vi "Periodic Tasks.vi"(8 "error in (no error)":errorcluster) -> ()   [LabVIEW 2012]
doc: "This VI runs in parallel to other tasks. It can contain as many user-defined periodic loops as you need. These can carry out PID or other sorts of timed response."
uses:
  <vilib>/Rock Robotics/SystemInterfaces/Utilities/FPGA_UtilitiesLED Source.ctl
  <vilib>/Rock Robotics/SystemInterfaces/Utilities/FPGA_UtilitiesLED State.ctl
  <vilib>/Rock Robotics/WPI/CAN/Jaguar/SubVIs/WPI_CANJaguar_StatusSelect.ctl
  <vilib>/addons/Kinect/Skeleton Vertex Index.ctl
  <vilib>/addons/Kinect/SkeletonVertexTrackState.ctl
  Robot Global Data.vi
  <vilib>/addons/control/pid/pid.llb/PID (DBL).vi
  <vilib>/Rock Robotics/WPI/Joystick/WPI_JoystickGetSetRefNum.vi
  <vilib>/addons/control/pid/NI_PID_pid.lvlib
panel:
  in  "Kinect Drive?":bool
  in  "Kinect?":bool
  in  "Constant":dbl=-0.02
  in  "Not PID?":bool=TRUE
  in  "PID gains":T1={"proportional gain (Kc)"=1.0, "integral time (Ti, min)"=0.01, "derivative time (Td, min)"=0.0} {"derivative time (Td, min)" format="%.3f"; "integral time (Ti, min)" format="%.3f"; "proportional gain (Kc)" format="%.3f"}
  in  "c":dbl
  in  "b":dbl
  in  "a":dbl
  in  "Set Shooter speed":dbl
  in  "Linear":bool=TRUE
  in  "m":dbl=0.059
  in  "b":dbl=-0.047
  in  "Straight Add":dbl=20.0
  in  "Spin":dbl=0.5
  out "output":dbl format="%.2f"
  out "Set Speed":dbl
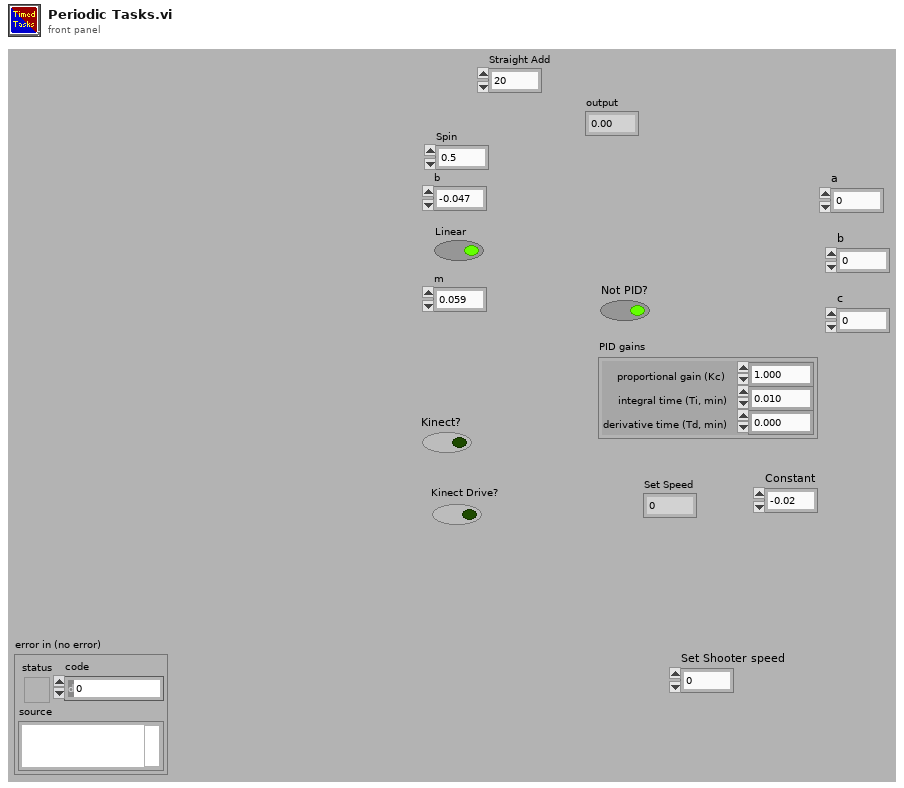
[diagram p1: front panel]
types:
  T1 = cluster{"proportional gain (Kc)":dbl, "integral time (Ti, min)":dbl, "derivative time (Td, min)":dbl}
  T2 = typedef "WPI_ServoDeviceRef.ctl" = cluster{"DeviceStatus":errorcluster, "Digital Module":T3, "PWM Channel":T4, "DeadBand":T5}
  T3 = typedef "FPGA_TypedefDigitalModule.ctl" = enum16{"Digital Module 1", "Digital Module 2"}
  T4 = typedef "FPGA_DIOPWMChannel.ctl" = enum8{"PWM 1", "PWM 2", "PWM 3", "PWM 4", "PWM 5", "PWM 6", "PWM 7", "PWM 8", "PWM 9", "PWM 10", "Invalid"}
  T5 = typedef "WPI_PWMDeadband.ctl" = cluster{"Name":string, "maxPositivePwm":i32, "minPositivePwm":i32, "centerPwm":i32, "maxNegativePwm":i32, "minNegativePwm":i32, "angularRange":u16}
  T6 = typedef "WPI_GyroDevRef.ctl" = cluster{"DevStatus":errorcluster, "Analog Module":T7, "Analog Channel":T8, "Offset":dbl, "Gain (VoltsPerDegree/Second)":dbl}
  T7 = typedef "FPGA_TypedefAnalogModule.ctl" = enum16{"Analog Module 1", "Analog Module 2"}
  T8 = typedef "FPGA_AIChannel.ctl" = enum8{"AI 1", "AI 2", "AI 3", "AI 4", "AI 5", "AI 6", "AI 7", "AI 8", "Invalid"}
  T9 = typedef "WPI_JoystickDevRef.ctl" = cluster{"Device":T10}
  T10 = typedef "WPI_JoystickDeviceEnum.ctl" = enum16{"USB 1", "USB 2", "USB 3", "USB 4", "Kinect 1", "Kinect 2"}
  T11 = typedef "WPI_MotorControlDeviceRef.ctl" = cluster{"DeviceStatus":errorcluster, "Type":enum16{"PWM", "CAN"}, "PWM":cluster{"Digital Module":T3, "PWM Channel":T4, "DeadBand":T5}, "CAN":cluster{"Device Number":u8, "Control Mode":T12, "Semaphore":T13, "Max Vout":dbl}, "Invert":bool, "TransformRef":T14, "InvTransformRef":T14}
  T12 = typedef "WPI_CANJaguar_ControlMode.ctl" = enum8{"Percent VBus", "Current", "Speed", "Position", "Voltage"}
  T13 = typedef "Semaphore RefNum" = refnum<k1>
  T14 = typedef "WPI_PWMTransform_ConPane.ctl" = refnum<vi>
  T15 = typedef "WPI_CANJaguar_StatusSelect.ctl" = enum16{"Output Percent VBus", "Output Voltage", "Bus Voltage", "Current", "Temperature", "Position", "Speed", "Limit Switches", "Faults", "Fault Counters", "Power Cycle"}
  T16 = typedef "Skeleton Vertex Index.ctl" = i32
  T17 = typedef "SkeletonVertexTrackState.ctl" = enum32{"NotTracked", "Inferred", "Tracked"}
  T18 = typedef "WPI_CANJaguar_Status.ctl" = cluster{"Output Percent VBus":dbl, "Output Voltage":dbl, "Bus Voltage":dbl, "Current":dbl, "Temperature":dbl, "Position":dbl, "Speed":dbl, "Limits":cluster{"Forward Limit":bool, "Reverse Limit":bool, "Forward Soft Limit":bool, "Reverse Soft Limit":bool, "Sticky Forward Limit":bool, "Sticky Reverse Limit":bool, "Sticky Forward Soft Limit":bool, "Sticky Reverse Soft Limit":bool}, "Faults":cluster{"Current Fault":bool, "Temperature Fault":bool, "Bus Voltage Fault":bool, "Gate Driver Fault":bool, "Comm Fault":bool}, "Fault Counters":cluster{"Current Faults":u8, "Temperature Faults":u8, "Bus Voltage Faults":u8, "Gate Driver Faults":u8, "Comm Faults":u8, "CAN Status":u8, "CAN RX Errors":u8, "CAN TX Errors":u8}, "Power Cycle":bool}
  T19 = cluster{cluster{"Left":dbl, "Top":dbl, "Right":dbl, "Bottom":dbl}, dbl[]}[]
  T20 = cluster{cluster{dbl, dbl, dbl}, cluster{"Right":dbl, "Left":dbl, "Bottom":dbl, "Top":dbl}}
  T21 = cluster{"Right":dbl, "Left":dbl, "Bottom":dbl, "Top":dbl}
  T22 = cluster{"axis 1 (x)":dbl, "axis 2 (y)":dbl, "axis 3 (throttle)":dbl, "axis 4":dbl, "axis 5":dbl, "axis 6":dbl}
  T23 = typedef "WPI_JoystickButtonState.ctl" = cluster{"Button 1":bool, "Button 2":bool, "Button 3":bool, "Button 4":bool, "Button 5":bool, "Button 6":bool, "Button 7":bool, "Button 8":bool, "Button 9":bool, "Button 10":bool, "Button 11":bool, "Button 12":bool}
  T24 = typedef "FPGA_UtilitiesLED State.ctl" = enum16{"Off", "On", "Toggle"}
  T25 = typedef "FPGA_UtilitiesLED Source.ctl" = enum16{"User LED", "FPGA LED"}
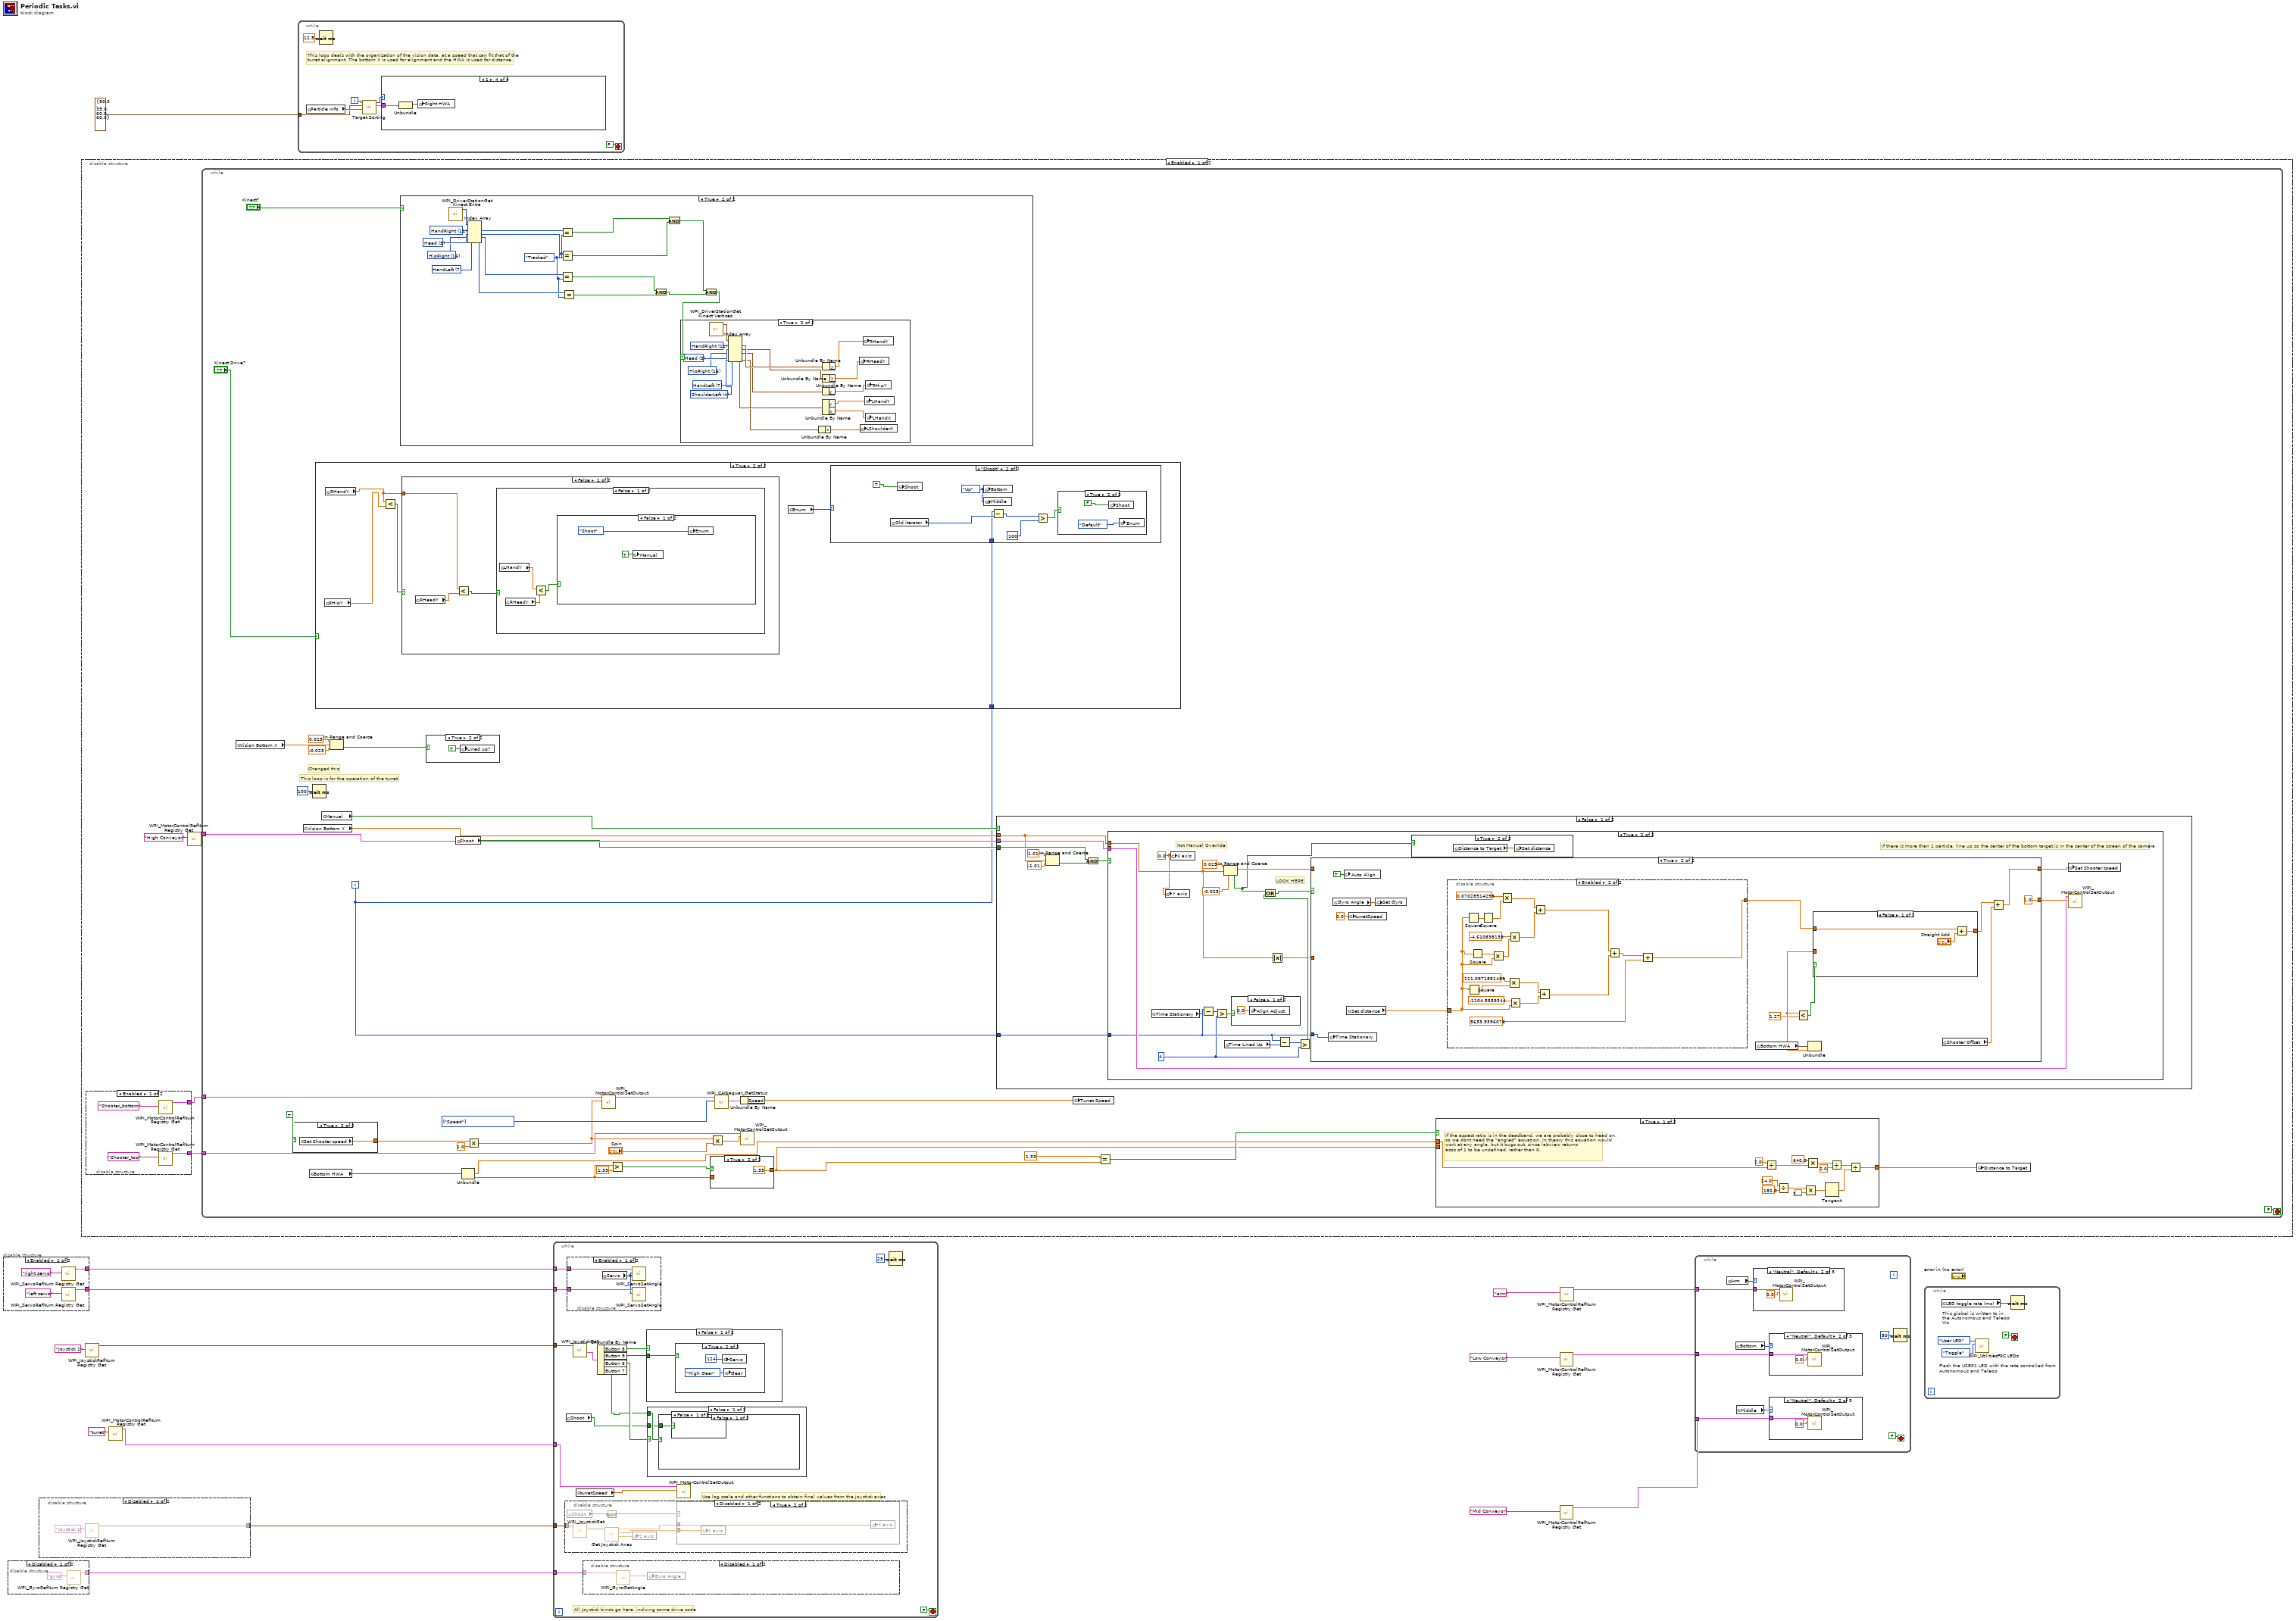
[diagram p0: block diagram]
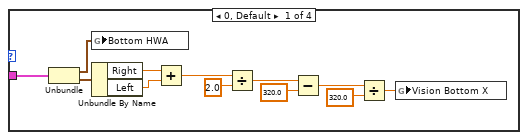
[diagram p3: hidden frame]
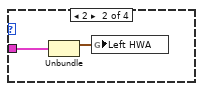
[diagram p4: hidden frame]
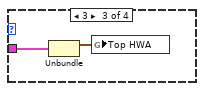
[diagram p5: hidden frame]
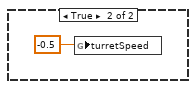
[diagram p11: hidden frame]
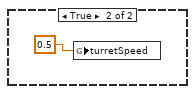
[diagram p12: hidden frame]
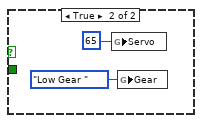
[diagram p15: hidden frame]
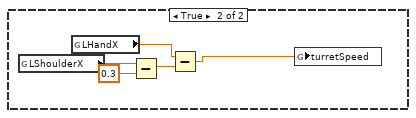
[diagram p19: hidden frame]
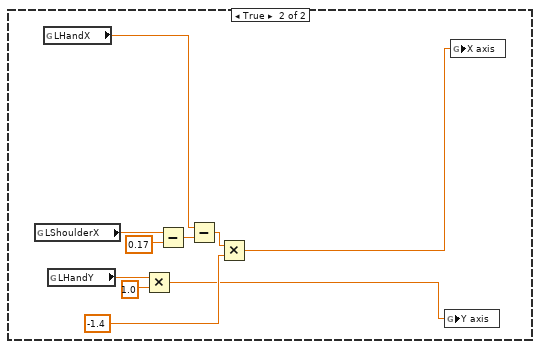
[diagram p20: hidden frame]
diagram:
  n1 = disable-structure shown="Enabled" {
    disable-tunnel: [w17 _] -> w9
    disable-tunnel: [w16 _] -> w8
    frame Enabled {
      n2 = call <vilib>:"WPI_ServoRefNum Registry Get.vi"("refnum name"="right servo") -> ("ServoDeviceRef"=w17:T2)  [unwired: 9 in, 1 out]
      n3 = call <vilib>:"WPI_ServoRefNum Registry Get.vi"("refnum name"="left servo") -> ("ServoDeviceRef"=w16:T2)  [unwired: 9 in, 1 out]
    }
    frame Disabled {
    }
  }
  n4 = disable-structure shown="Disabled" {
    disable-tunnel: [w21 _] -> w11
    frame Disabled {
      n5 = call <vilib>:"WPI_GyroRefNum Registry Get.vi"("refnum name"="gyro") -> ("GyroDevRef"=w21:T6)  [unwired: 9 in, 1 out]
    }
    frame Enabled {
    }
  }
  n6 = disable-structure shown="Disabled" {
    disable-tunnel: [w22 _] -> w12
    frame Disabled {
      n7 = call <vilib>:"WPI_JoystickRefNum Registry Get.vi"("refnum name"="Joystick 1") -> ("JoystickDevRef"=w22:T9)  [unwired: 9 in, 1 out]
    }
    frame Enabled {
    }
  }
  n8 = disable-structure shown="Enabled" {
    frame Enabled {
      n9 = disable-structure shown="Enabled" {
        disable-tunnel: [w31 _] -> w27
        disable-tunnel: [w30 _] -> w26
        frame Enabled {
          n10 = call <vilib>:"WPI_MotorControlRefNum Registry Get.vi"("refnum name"="Shooter_bottom") -> ("MotorControlDevRef"=w30:T11)  [unwired: 9 in, 1 out]
          n11 = call <vilib>:"WPI_MotorControlRefNum Registry Get.vi"("refnum name"="Shooter_top") -> ("MotorControlDevRef"=w31:T11)  [unwired: 9 in, 1 out]
        }
        frame Disabled {
        }
      }
      n12 = call <vilib>:"WPI_MotorControlRefNum Registry Get.vi"("refnum name"="High Conveyor") -> ("MotorControlDevRef"=w24:T11)  [unwired: 9 in, 1 out]
      n13 = while {
        tunnel: w27 -> [w63]
        tunnel: w26 -> [w62]
        tunnel: w24 -> [w39]
        i -> [w33]
        stop <- FALSE stop-if-true
        w58 = T15[] [enum."Speed"] items=["Output Percent VBus", "Output Voltage", "Bus Voltage", "Current", "Temperature", "Position", "Speed", "Limit Switches", "Faults", "Fault Counters", "Power Cycle"] ("Status Select")
        # "Changed this"
        # "This loop is for the operation of the turret."
        n14 = global read "Robot Global Data.vi" "Vision Bottom X"() -> (w43:dbl)
        n15 = case shown="True" TRUE {
          tunnel: ["Set Shooter speed" w145] -> w55
          frame False {
          }
          frame True {
            n16 = global read "Robot Global Data.vi" "Set Shooter speed"() -> (w145:dbl)
          }
        }
        n17 = global read "Robot Global Data.vi" "Vision Bottom X"() -> (w37:dbl)
        n18 = global read "Robot Global Data.vi" "Bottom HWA"() -> (w50:cluster{dbl, dbl, dbl})
        n19 = Wait (ms)(milliseconds to wait=u32 100) -> ()  [unwired: 1 out]
        n20 = case shown="True" "Kinect Drive?" {
          tunnel: w33 -> [_ w69]
          frame False {
          }
          frame True {
            n21 = global read "Robot Global Data.vi" "RHipY"() -> (w68:dbl)
            n22 = global read "Robot Global Data.vi" "RHandY"() -> (w66:dbl)
            n23 = Less?(x=w66, y=w68) -> (x < y?=w67:bool)
            n24 = case shown="False" w67 {
              tunnel: w66 -> [w73 _]
              frame False {
                n25 = global read "Robot Global Data.vi" "RHeadY"() -> (w72:dbl)
                n26 = Less?(x=w73, y=w72) -> (x < y?=w71:bool)
                n27 = case shown="False" w71 {
                  frame False {
                    n28 = global read "Robot Global Data.vi" "LHandY"() -> (w75:dbl)
                    n29 = global read "Robot Global Data.vi" "RHeadY"() -> (w74:dbl)
                    n30 = Less?(x=w75, y=w74) -> (x < y?=w76:bool)
                    n31 = case shown="False" w76 {
                      frame False {
                        n32 = global write "Robot Global Data.vi" "Manual"(TRUE ("Manual")) -> ()
                        n33 = global write "Robot Global Data.vi" "Enum"(enum16{"Default", "Shoot"}."Shoot" ("Enum")) -> ()
                      }
                      frame True {
                        n34 = global read "Robot Global Data.vi" "LShoulderX"() -> (w83:dbl)
                        n35 = global read "Robot Global Data.vi" "LHandX"() -> (w82:dbl)
                        n36 = Subtract(x=w83, y=0.3) -> (x-y=w80:dbl)
                        n37 = Subtract(x=w82, y=w80) -> (x-y=w81:dbl)
                        n38 = global write "Robot Global Data.vi" "turretSpeed"(w81) -> ()
                      }
                    }
                  }
                  frame True {
                    n39 = global read "Robot Global Data.vi" "LShoulderX"() -> (w87:dbl)
                    n40 = global read "Robot Global Data.vi" "LHandX"() -> (w93:dbl)
                    n41 = global read "Robot Global Data.vi" "LHandY"() -> (w92:dbl)
                    n42 = Multiply(x=w92, y=1.0) -> (x*y=w90:dbl)
                    n43 = Subtract(x=w87, y=0.17 ("x")) -> (x-y=w85:dbl)
                    n44 = Subtract(x=w93, y=w85) -> (x-y=w88:dbl)
                    n45 = Multiply(x=w88, y=-1.4) -> (x*y=w86:dbl)
                    n46 = global write "Robot Global Data.vi" "Y axis"(w90) -> ()
                    n47 = global write "Robot Global Data.vi" "X axis"(w86) -> ()
                  }
                }
              }
              frame True {
                w94 = 0.0 ("X axis")
                n48 = global write "Robot Global Data.vi" "X axis"(w94) -> ()
                n49 = global write "Robot Global Data.vi" "Y axis"(0.0 ("Y axis")) -> ()
                n50 = global write "Robot Global Data.vi" "Shoot"(FALSE) -> ()
                n51 = global write "Robot Global Data.vi" "turretSpeed"(w94) -> ()
                n52 = global write "Robot Global Data.vi" "Enum"(enum16{"Default", "Shoot"}."Default" ("Enum")) -> ()
              }
            }
            n53 = global read "Robot Global Data.vi" "Enum"() -> (w70:enum16{"Default", "Shoot"})
            n54 = case shown="\"Shoot\"" w70 {
              tunnel: w69 -> [w100 w103]
              frame "Default", Default {
                w99 = enum16{"Up", "Neutral", "Down"}."Neutral" ("Bottom")
                n55 = global write "Robot Global Data.vi" "Set Shooter speed"(0.0 ("Set Shooter speed")) -> ()
                n56 = global write "Robot Global Data.vi" "Old iterator"(w100) -> ()
                n57 = global write "Robot Global Data.vi" "Bottom"(w99) -> ()
                n58 = global write "Robot Global Data.vi" "Bottom"(w99) -> ()
              }
              frame "Shoot" {
                w101 = enum16{"Up", "Neutral", "Down"}."Up" ("Bottom")
                n59 = global read "Robot Global Data.vi" "Old iterator"() -> (w104:i8)
                n60 = global write "Robot Global Data.vi" "Shoot"(TRUE) -> ()
                n61 = global write "Robot Global Data.vi" "Bottom"(w101) -> ()
                n62 = global write "Robot Global Data.vi" "Middle"(w101) -> ()
                n63 = Subtract(x=w103, y=w104) -> (x-y=w102:i32)
                n64 = Greater?(x=w102, y=u32 100 ("milliseconds to wait")) -> (0:w105:bool)
                n65 = case shown="True" w105 {
                  frame False {
                  }
                  frame True {
                    n66 = global write "Robot Global Data.vi" "Shoot"(FALSE) -> ()
                    n67 = global write "Robot Global Data.vi" "Enum"(enum16{"Default", "Shoot"}."Default" ("Enum")) -> ()
                  }
                }
              }
            }
          }
        }
        n68 = global read "Robot Global Data.vi" "Manual"() -> (w35:bool)
        n69 = In Range and Coerce(upper limit=0.025, x=w43, lower limit=-0.025) -> (In Range?=w40:bool)  [unwired: 1 out]
        n70 = case shown="True" "Kinect?" {
          frame False {
          }
          frame True {
            w118 = T16 7 items=["HipCenter", "Spine", "ShoulderCenter", "Head", "ShoulderLeft", "ElbowLeft", "WristLeft", "HandLeft", "ShoulderRight", "ElbowRight", "WristRight", "HandRight", "HipLeft", "KneeLeft", "AnkleLeft", "FootLeft", "HipRight", "KneeRight", "AnkleRight", "FootRight"] ("Skeleton Joints")
            w119 = T16 16 items=["HipCenter", "Spine", "ShoulderCenter", "Head", "ShoulderLeft", "ElbowLeft", "WristLeft", "HandLeft", "ShoulderRight", "ElbowRight", "WristRight", "HandRight", "HipLeft", "KneeLeft", "AnkleLeft", "FootLeft", "HipRight", "KneeRight", "AnkleRight", "FootRight"] ("Skeleton Joints")
            w123 = T16 3 items=["HipCenter", "Spine", "ShoulderCenter", "Head", "ShoulderLeft", "ElbowLeft", "WristLeft", "HandLeft", "ShoulderRight", "ElbowRight", "WristRight", "HandRight", "HipLeft", "KneeLeft", "AnkleLeft", "FootLeft", "HipRight", "KneeRight", "AnkleRight", "FootRight"] ("Skeleton Joints")
            w115 = SkeletonVertexTrackState."Tracked" ("element")
            w125 = T16 11 items=["HipCenter", "Spine", "ShoulderCenter", "Head", "ShoulderLeft", "ElbowLeft", "WristLeft", "HandLeft", "ShoulderRight", "ElbowRight", "WristRight", "HandRight", "HipLeft", "KneeLeft", "AnkleLeft", "FootLeft", "HipRight", "KneeRight", "AnkleRight", "FootRight"] ("Skeleton Joints")
            n71 = call <vilib>:"WPI_DriverStationGet Kinect Extra.vi"() -> ("Skeleton Tracking State"=w126:T17[])  [unwired: 7 in, 4 out]
            n72 = Index Array(array=w126, index #1=w125, index #2=w123, index #3=w119, index #4=w118) -> (element #1=w124:T17, element #2=w122:T17, element #3=w117:T17, element #4=w116:T17)
            n73 = Equal?(x=w124, y=w115) -> (x = y?=w121:bool)
            n74 = Equal?(x=w115, y=w122) -> (x = y?=w120:bool)
            n75 = Equal?(x=w117, y=w115) -> (x = y?=w114:bool)
            n76 = Equal?(x=w116, y=w115) -> (x = y?=w113:bool)
            n77 = And(x=w114, y=w113) -> (x .and. y?=w112:bool)
            n78 = And(x=w121, y=w120) -> (x .and. y?=w111:bool)
            n79 = And(x=w111, y=w112) -> (x .and. y?=w110:bool)
            n80 = case shown="True" w110 {
              frame False {
                (unwired) 0.0
              }
              frame True {
                w129 = T16 4 items=["HipCenter", "Spine", "ShoulderCenter", "Head", "ShoulderLeft", "ElbowLeft", "WristLeft", "HandLeft", "ShoulderRight", "ElbowRight", "WristRight", "HandRight", "HipLeft", "KneeLeft", "AnkleLeft", "FootLeft", "HipRight", "KneeRight", "AnkleRight", "FootRight"] ("Skeleton Joints")
                w139 = T16 7 items=["HipCenter", "Spine", "ShoulderCenter", "Head", "ShoulderLeft", "ElbowLeft", "WristLeft", "HandLeft", "ShoulderRight", "ElbowRight", "WristRight", "HandRight", "HipLeft", "KneeLeft", "AnkleLeft", "FootLeft", "HipRight", "KneeRight", "AnkleRight", "FootRight"] ("Skeleton Joints")
                w140 = T16 16 items=["HipCenter", "Spine", "ShoulderCenter", "Head", "ShoulderLeft", "ElbowLeft", "WristLeft", "HandLeft", "ShoulderRight", "ElbowRight", "WristRight", "HandRight", "HipLeft", "KneeLeft", "AnkleLeft", "FootLeft", "HipRight", "KneeRight", "AnkleRight", "FootRight"] ("Skeleton Joints")
                w141 = T16 3 items=["HipCenter", "Spine", "ShoulderCenter", "Head", "ShoulderLeft", "ElbowLeft", "WristLeft", "HandLeft", "ShoulderRight", "ElbowRight", "WristRight", "HandRight", "HipLeft", "KneeLeft", "AnkleLeft", "FootLeft", "HipRight", "KneeRight", "AnkleRight", "FootRight"] ("Skeleton Joints")
                w142 = T16 11 items=["HipCenter", "Spine", "ShoulderCenter", "Head", "ShoulderLeft", "ElbowLeft", "WristLeft", "HandLeft", "ShoulderRight", "ElbowRight", "WristRight", "HandRight", "HipLeft", "KneeLeft", "AnkleLeft", "FootLeft", "HipRight", "KneeRight", "AnkleRight", "FootRight"] ("Skeleton Joints")
                n81 = call <vilib>:"WPI_DriverStationGet Kinect Vertices.vi"() -> ("Skeleton Vertices"=w143:cluster{"x":sgl, "y":sgl, "z":sgl}[])  [unwired: 10 in, 1 out]
                n82 = Index Array(array=w143, index #1=w142, index #2=w141, index #3=w140, index #4=w139, index #5=w129) -> (element #1=w138:cluster{"x":sgl, "y":sgl, "z":sgl}, element #2=w137:cluster{"x":sgl, "y":sgl, "z":sgl}, element #3=w136:cluster{"x":sgl, "y":sgl, "z":sgl}, element #4=w135:cluster{"x":sgl, "y":sgl, "z":sgl}, element #5=w127:cluster{"x":sgl, "y":sgl, "z":sgl})
                n83 = Unbundle By Name(w127) -> ("x"=w128:sgl)
                n84 = Unbundle By Name(w136) -> ("y"=w132:sgl)
                n85 = Unbundle By Name(w135) -> ("y"=w131:sgl, "x"=w130:sgl)
                n86 = Unbundle By Name(w138) -> ("y"=w134:sgl)
                n87 = Unbundle By Name(w137) -> ("y"=w133:sgl)
                n88 = global write "Robot Global Data.vi" "RHeadY"(w133) -> ()
                n89 = global write "Robot Global Data.vi" "LShoulderX"(w128) -> ()
                n90 = global write "Robot Global Data.vi" "RHandY"(w134) -> ()
                n91 = global write "Robot Global Data.vi" "LHandY"(w131) -> ()
                n92 = global write "Robot Global Data.vi" "RHipY"(w132) -> ()
                n93 = global write "Robot Global Data.vi" "LHandX"(w130) -> ()
              }
            }
          }
        }
        n94 = case shown="True" w40 {
          frame False {
            n95 = global write "Robot Global Data.vi" "Lined up?"(FALSE ("Lined up?")) -> ()
          }
          frame True {
            n96 = global write "Robot Global Data.vi" "Lined up?"(TRUE ("Lined up?")) -> ()
          }
        }
        n97 = global read "Robot Global Data.vi" "Shoot"() -> (w38:bool)
        n98 = Unbundle(w50) -> (w52:dbl, w44:dbl)  [unwired: 1 out]
        n99 = Multiply(x=w55, y=1.0) -> (x*y=w56:dbl)
        n100 = call <vilib>:"WPI_MotorControlSetOutput.vi"("Output"=w56, "MotorControlDevRef"=w62) -> ("MotorControlDevRef"=w59:T11)  [unwired: 7 in, 2 out]
        n101 = Greater?(x=w44, y=1.33) -> (0:w48:bool)
        n102 = case shown="True" w48 {
          tunnel: [w148 1.33 ("y")] -> w45
          tunnel: w44 -> [w148 _]
          frame False {
          }
          frame True {
          }
        }
        n103 = Multiply(x=w56, y="Spin") -> (x*y=w54:dbl)
        n104 = call <vilib>:"WPI_CANJaguar_GetStatus.vi"("Status Select"=w58, "CAN Jaguar Ref"=w59) -> ("Status"=w60:T18)  [unwired: 7 in, 2 out]
        n105 = Unbundle By Name(w60) -> ("Speed"=w61:dbl)
        n106 = call <vilib>:"WPI_MotorControlSetOutput.vi"("Output"=w54, "MotorControlDevRef"=w63) -> ()  [unwired: 7 in, 3 out]
        n107 = case shown="False" w35 {
          tunnel: w39 -> [w196 w340]
          tunnel: w38 -> [w195 _]
          tunnel: w37 -> [w194 _]
          tunnel: w33 -> [w189 _]
          frame False {
            n108 = In Range and Coerce(upper limit=1.01, x=w194, lower limit=-1.01) -> (In Range?=w190:bool)  [unwired: 1 out]
            n109 = And(x=w195, y=w190) -> (x .and. y?=w191:bool)
            n110 = case shown="True" w191 {
              tunnel: w196 -> [w200 w219]
              tunnel: w194 -> [_ w213]
              tunnel: w189 -> [w197 w208]
              frame False {
                n111 = global write "Robot Global Data.vi" "Time Stationary"(w197) -> ()
                n112 = global write "Robot Global Data.vi" "Time Lined Up"(w197) -> ()
                n113 = call <vilib>:"WPI_MotorControlSetOutput.vi"("Output"=0.0, "MotorControlDevRef"=w200) -> ()  [unwired: 7 in, 3 out]
                n114 = global write "Robot Global Data.vi" "Set Shooter speed"(0.0 ("Set Shooter speed")) -> ()
              }
              frame True {
                w202 = 0.0 ("X axis")
                w205 = 4 ("y")
                # "LOOK HERE"
                # "If there is more than 1 particle, line up so the center of the bottom target is in the center of the screen of the camera"
                # "Not Manual Override"
                n115 = global read "Robot Global Data.vi" "Time Stationary"() -> (w207:i32)
                n116 = global write "Robot Global Data.vi" "Y axis"(w202) -> ()
                n117 = global write "Robot Global Data.vi" "X axis"(w202) -> ()
                n118 = Subtract(x=w208, y=w207) -> (x-y=w206:i32)
                n119 = Greater?(x=w206, y=w205) -> (0:w204:bool)
                n120 = In Range and Coerce(upper limit=0.025, x=w213, lower limit=-0.025) -> (coerced(x)=w216:dbl, In Range?=w209:bool)
                n121 = global read "Robot Global Data.vi" "Time Lined Up"() -> (w212:i32)
                n122 = case shown="False" w204 {
                  frame False {
                    n123 = global write "Robot Global Data.vi" "Align Adjust"(0.0 ("Align Adjust")) -> ()
                  }
                  frame True {
                    n124 = global write "Robot Global Data.vi" "Align Adjust"(0.05 ("Align Adjust")) -> ()
                  }
                }
                n125 = Absolute Value(x=w213) -> (abs(x)=w201:dbl)
                n126 = Subtract(x=w208, y=w212) -> (x-y=w211:i32)
                n127 = Greater?(x=w211, y=w205) -> (0:w210:bool)
                n128 = Or(x=w209, y=w210) -> (x .or. y?=w203:bool)
                n129 = case shown="True" w203 {
                  tunnel: w216 -> [w234 _]
                  tunnel: [w242 w281] -> w215
                  tunnel: [w242 1.0 ("Output")] -> w214
                  tunnel: w201 -> [w241 _]
                  tunnel: w208 -> [w232 w278]
                  frame False {
                    w242 = 0.0
                    n130 = global write "Robot Global Data.vi" "Time Lined Up"(w232) -> ()
                    n131 = feedback-in #1(w234) -> ()
                    n132 = feedback #1() -> (w235:dbl)  [unwired: 1 in]
                    n133 = Sign(1:w234) -> (0:w236:dbl)
                    n134 = case shown="True" "Not PID?" {
                      tunnel: w241 -> [w250 w254]
                      tunnel: [w247 w253] -> w240
                      tunnel: w236 -> [_ w252]
                      frame False {
                        n135 = call-poly <vilib>:"PID.vi"("PID gains"="PID gains", "process variable"=w250, "setpoint"=0.0) -> ("output"=w247:dbl)  [unwired: 7 in, 1 out]
                      }
                      frame True {
                        n136 = case shown="False" "Linear" {
                          tunnel: w254 -> [w258 w274]
                          tunnel: [w261 w271] -> w253
                          tunnel: w252 -> [_ w270]
                          frame False {
                            n137 = Square(x=w258) -> (x^2=w263:dbl)
                            n138 = Multiply(x=w263, y="a") -> (x*y=w259:dbl)
                            n139 = Multiply(x="b", y=w258) -> (x*y=w257:dbl)
                            n140 = Add(x=w257, y=w259) -> (x+y=w256:dbl)
                            n141 = Add(x="c", y=w256) -> (x+y=w261:dbl)
                          }
                          frame True {
                            n142 = Divide(x="m", y=1.0) -> (x/y=w265:dbl)
                            n143 = Divide(x="b", y=1.0) -> (x/y=w269:dbl)
                            n144 = Multiply(x=w270, y=w265) -> (x*y=w273:dbl)
                            n145 = Multiply(x=w274, y=w269) -> (x*y=w272:dbl)
                            n146 = Add(x=w273, y=w272) -> (x+y=w271:dbl)
                          }
                        }
                      }
                    }
                    n147 = Equal?(x=w235, y=w234) -> (x = y?=w233:bool)
                    n148 = case shown="False" w233 {
                      tunnel: w232 -> [w275 _]
                      frame False {
                        n149 = global write "Robot Global Data.vi" "Time Stationary"(w275) -> ()
                      }
                      frame True {
                      }
                    }
                    n150 = Absolute Value(x=w240) -> (abs(x)=w239:dbl)
                    n151 = Add(x="Constant", y=w239) -> (x+y=w228:dbl)
                    n152 = In Range and Coerce(upper limit=0.22, x=w228, lower limit=0.065) -> (coerced(x)=w230:dbl)  [unwired: 1 out]
                    n153 = global write "Robot Global Data.vi" "Auto Align"(FALSE ("Auto Align")) -> ()
                    n154 = Multiply(x=w236, y=w230) -> (x*y=w224:dbl)
                    n155 = Less?(x=w224, y=0.0) -> (x < y?=w225:bool)
                    n156 = case shown="False" w225 {
                      tunnel: w224 -> [w243 w245]
                      tunnel: [w243 w244] -> w223
                      frame False {
                      }
                      frame True {
                        n157 = Subtract(x=w245, y=0.01) -> (x-y=w244:dbl)
                      }
                    }
                    "output" <- w223
                    n158 = global write "Robot Global Data.vi" "turretSpeed"(w223) -> ()
                  }
                  frame True {
                    n159 = global write "Robot Global Data.vi" "Time Stationary"(w278) -> ()
                    n160 = global read "Robot Global Data.vi" "Gyro Angle"() -> (w279:dbl)
                    n161 = global write "Robot Global Data.vi" "Auto Align"(TRUE ("Auto Align")) -> ()
                    n162 = global read "Robot Global Data.vi" "Set distance"() -> (w282:dbl)
                    n163 = global write "Robot Global Data.vi" "turretSpeed"(0.0 ("turretSpeed")) -> ()
                    n164 = global write "Robot Global Data.vi" "Set Gyro"(w279) -> ()
                    n165 = disable-structure shown="Enabled" {
                      disable-tunnel: [w292 w303] -> w287
                      disable-tunnel: w282 -> [w291 w312]
                      frame Disabled {
                        n166 = Square(x=w291) -> (x^2=w300:dbl)
                        n167 = Multiply(x=w300, y=w291) -> (x*y=w290:dbl)
                        n168 = Multiply(x=0.24778100093141, y=w290) -> (x*y=w301:dbl)
                        n169 = Multiply(x=w300, y=11.172728810856) -> (x*y=w298:dbl)
                        n170 = Subtract(x=w301, y=w298) -> (x-y=w296:dbl)
                        n171 = Multiply(x=w291, y=203.71864672698) -> (x*y=w297:dbl)
                        n172 = Add(x=w296, y=w297) -> (x+y=w294:dbl)
                        n173 = Add(x=w294, y=710.6891050634) -> (x+y=w292:dbl)
                      }
                      frame Enabled {
                        n174 = Square(x=w312) -> (x^2=w320:dbl)
                        n175 = Square(x=w312) -> (x^2=w314:dbl)
                        n176 = Square(x=w312) -> (x^2=w317:dbl)
                        n177 = Square(x=w320) -> (x^2=w319:dbl)
                        n178 = Multiply(x=w317, y=w312) -> (x*y=w316:dbl)
                        n179 = Multiply(x=0.07028514299 ("y"), y=w319) -> (x*y=w311:dbl)
                        n180 = Multiply(x=111.0971851489 ("y"), y=w314) -> (x*y=w309:dbl)
                        n181 = Multiply(x=-4.610838138 ("y"), y=w316) -> (x*y=w310:dbl)
                        n182 = Multiply(x=-1104.5559344 ("y"), y=w312) -> (x*y=w308:dbl)
                        n183 = Add(x=w311, y=w310) -> (x+y=w307:dbl)
                        n184 = Add(x=w309, y=w308) -> (x+y=w306:dbl)
                        n185 = Add(x=w307, y=w306) -> (x+y=w304:dbl)
                        n186 = Add(x=w304, y=5633.9396076) -> (x+y=w303:dbl)
                      }
                    }
                    n187 = global read "Robot Global Data.vi" "Bottom HWA"() -> (w288:cluster{dbl, dbl, dbl})
                    n188 = Unbundle(w288) -> (w284:dbl)  [unwired: 2 out]
                    n189 = Less?(x=w284, y=1.27) -> (x < y?=w283:bool)
                    n190 = case shown="False" w283 {
                      tunnel: w284 -> [_ w335]
                      tunnel: w287 -> [w324 w327]
                      tunnel: [w323 w325] -> w286
                      frame False {
                        n191 = Add(x=w324, y="Straight Add") -> (x+y=w323:dbl)
                      }
                      frame True {
                        n192 = Subtract(x=1.33, y=w335) -> (x-y=w329:dbl)
                        n193 = Square(x=w329) -> (x^2=w333:dbl)
                        n194 = Multiply(x=432.52595155723, y=w333) -> (x*y=w331:dbl)
                        n195 = Multiply(x=w329, y=438.47058823534) -> (x*y=w330:dbl)
                        n196 = Add(x=w331, y=w330) -> (x+y=w326:dbl)
                        n197 = Subtract(x=w327, y=w326) -> (x-y=w325:dbl)
                      }
                    }
                    n198 = global read "Robot Global Data.vi" "Shooter Offset"() -> (w280:dbl)
                    n199 = Add(x=w286, y=w280) -> (x+y=w281:dbl)
                  }
                }
                n200 = case shown="True" w209 {
                  frame False {
                  }
                  frame True {
                    n201 = global read "Robot Global Data.vi" "Distance to Target"() -> (w222:dbl)
                    n202 = global write "Robot Global Data.vi" "Set distance"(w222) -> ()
                  }
                }
                n203 = global write "Robot Global Data.vi" "Set Shooter speed"(w215) -> ()
                n204 = call <vilib>:"WPI_MotorControlSetOutput.vi"("Output"=w214, "MotorControlDevRef"=w219) -> ()  [unwired: 7 in, 3 out]
              }
            }
          }
          frame True {
            n205 = global read "Robot Global Data.vi" "Shoot"() -> (w337:bool)
            n206 = case shown="True" w337 {
              tunnel: w340 -> [w343 w346]
              tunnel: [0.0 ("x") w347] -> _
              tunnel: [w343 w346] -> w339
              tunnel: [0.0 ("Output") 1.0 ("Output")] -> w338
              frame False {
              }
              frame True {
                w344 = 0.0 ("X axis")
                n207 = global write "Robot Global Data.vi" "Y axis"(w344) -> ()
                n208 = global write "Robot Global Data.vi" "X axis"(w344) -> ()
                n209 = global read "Robot Global Data.vi" "Shooter"() -> (w347:dbl)
                "Set Speed" <- w347
              }
            }
            n210 = call <vilib>:"WPI_MotorControlSetOutput.vi"("Output"=w338, "MotorControlDevRef"=w339) -> ()  [unwired: 7 in, 3 out]
            n211 = global write "Robot Global Data.vi" "Set Shooter speed"(500.0 ("Set Shooter speed")) -> ()
          }
        }
        n212 = global write "Robot Global Data.vi" "Turret Speed"(w61) -> ()
        n213 = Equal?(x=1.33 ("upper limit"), y=w45) -> (x = y?=w46:bool)
        n214 = case shown="True" w46 {
          tunnel: w52 -> [w156 w183]
          tunnel: w45 -> [_ w166]
          tunnel: [w155 w164] -> w51
          frame True {
            # "If the aspect ratio is in the deadband, we are probably close to head on, so we dont need the \"angled\" equation. In theory this equation would work at any angle, but it bugs out, since labview returns\nacos of 1 to be undefined, rather than 0."
            n215 = Divide(x=2.0 ("Target Width (ft)"), y=w156) -> (x/y=w161:dbl)
            n216 = Divide(x=24.0, y=180.0) -> (x/y=w152:dbl)
            n217 = Multiply(x=w152, y=3.141592653589793) -> (x*y=w151:dbl)
            n218 = Multiply(x=640.0 ("X Image Resolution"), y=w161) -> (x*y=w160:dbl)
            n219 = Tangent(1:w151) -> (0:w157:dbl)
            n220 = Divide(x=w160, y=2.0) -> (x/y=w158:dbl)
            n221 = Divide(x=w158, y=w157) -> (x/y=w155:dbl)
          }
          frame False {
            # "This function converts Aspect Ratio to Angle, Angle to  Width Offset, and the Offset to Distance"
            n222 = Divide(x=w166, y=1.33) -> (x/y=w176:dbl)
            n223 = Inverse Cosine(1:w176) -> (0:w174:dbl)
            n224 = expression code="(x/pi)*180.0" ("radians to degrees")(w174) -> (w170:dbl)
            n225 = Divide(x=133.0, y=122.0) -> (x/y=w171:dbl)
            n226 = Multiply(x=w171, y=w170) -> (x*y=w169:dbl)
            n227 = Power Of X(1:w169, 2:1.02 ("y")) -> (0:w167:dbl)
            n228 = Subtract(x=w167, y=73.0) -> (x-y=w186:dbl)
            n229 = Divide(x=-3.1, y=w186) -> (x/y=w185:dbl)
            n230 = Add(x=w185, y=0.833) -> (x+y=w182:dbl)
            n231 = expression code="(x/180.0)*pi" "degrees to radians"(24.0 ("x")) -> (w165:dbl)
            n232 = Multiply(x=w182, y=w183) -> (x*y=w180:dbl)
            n233 = Tangent(1:w165) -> (0:w179:dbl)
            n234 = Multiply(x=w180, y=w179) -> (x*y=w178:dbl)
            n235 = Divide(x=640.0, y=w178) -> (x/y=w164:dbl)
          }
        }
        n236 = global write "Robot Global Data.vi" "Distance to Target"(w51) -> ()
      }
    }
    frame Disabled {
    }
  }
  n237 = call <vilib>:"WPI_JoystickRefNum Registry Get.vi"("refnum name"="Joystick 1") -> ("JoystickDevRef"=w10:T9)  [unwired: 1 in, 9 out]
  n238 = call <vilib>:"WPI_MotorControlRefNum Registry Get.vi"("refnum name"="turret") -> ("MotorControlDevRef"=w2:T11)  [unwired: 9 in, 1 out]
  n239 = while {
    tunnel: cluster{dbl, dbl, dbl, dbl} {80.0, 35.0, 60.0, 60.0} ("Cluster") -> [w353]
    i -> [w352]
    stop <- FALSE stop-if-true
    # "This loop deals with the organization of the vision data, at a speed that can fit that of the \nturret alignment. The bottom X is used for alignment and the HWA is used for distance."
    n240 = global read "Robot Global Data.vi" "Particle Info"() -> (w354:T19)
    n241 = Wait (ms)(milliseconds to wait=12.5) -> ()  [unwired: 1 out]
    n242 = call "Target Sorting.vi"("Particle Info"=w354, "Particle scores for comparison"=w353, "Iterator"=w352) -> ("output cluster"=w349:T20, "Numeric out"=w350:i32)  [unwired: 4 in, 3 out]
    n243 = case shown="1" w350 {
      tunnel: w349 -> [w366 w368 w370 w372]
      frame 0, Default {
        n244 = Unbundle(w366) -> (w355:cluster{dbl, dbl, dbl}, w357:T21)
        n245 = global write "Robot Global Data.vi" "Bottom HWA"(w355) -> ()
        n246 = Unbundle By Name(w357) -> ("Right"=w358:dbl, "Left"=w359:dbl)
        n247 = Add(x=w358, y=w359) -> (x+y=w360:dbl)
        n248 = Divide(x=w360, y=2.0) -> (x/y=w362:dbl)
        n249 = Subtract(x=w362, y=320.0) -> (x-y=w364:dbl)
        n250 = Divide(x=w364, y=320.0) -> (x/y=w356:dbl)
        n251 = global write "Robot Global Data.vi" "Vision Bottom X"(w356) -> ()
      }
      frame 2 {
        n252 = Unbundle(w368) -> (w367:cluster{dbl, dbl, dbl})  [unwired: 1 out]
        n253 = global write "Robot Global Data.vi" "Left HWA"(w367) -> ()
      }
      frame 3 {
        n254 = Unbundle(w370) -> (w369:cluster{dbl, dbl, dbl})  [unwired: 1 out]
        n255 = global write "Robot Global Data.vi" "Top HWA"(w369) -> ()
      }
      frame 1 {
        n256 = Unbundle(w372) -> (w371:cluster{dbl, dbl, dbl})  [unwired: 1 out]
        n257 = global write "Robot Global Data.vi" "Right HWA"(w371) -> ()
      }
    }
  }
  n258 = while {
    tunnel: w12 -> [w385]
    tunnel: w11 -> [w384]
    tunnel: w10 -> [w383]
    tunnel: w9 -> [w382]
    tunnel: w8 -> [w381]
    tunnel: w2 -> [w376]
    stop <- FALSE stop-if-true
    # "Use log scale and other functions to obtain final values from the joystick axes"
    # "All Joystick binds go here, incluing some drive code"
    n259 = disable-structure shown="Disabled" {
      disable-tunnel: w385 -> [w392 _]
      frame Disabled {
        n260 = global read "Robot Global Data.vi" "Shoot"() -> (w389:bool)
        n261 = call <vilib>:"WPI_JoystickGet.vi"("JoystickDevRef"=w392) -> ("Axes"=w391:T22)  [unwired: 1 in, 5 out]
        n262 = Not(x=w389) -> (.not. x?=w388:bool)
        n263 = call "Get Joystick Axes.vi"("Axes"=w391) -> ("Numeric"=w390:dbl, "joystick out"=w393:dbl, "joystick out 2"=w394:dbl)  [unwired: 8 in]
        n264 = global write "Robot Global Data.vi" "Z axis"(w390) -> ()
        n265 = case shown="True" w388 {
          tunnel: w394 -> [_ w396]
          tunnel: w393 -> [_ w395]
          frame False {
          }
          frame True {
            n266 = global write "Robot Global Data.vi" "Y axis"(w395) -> ()
            n267 = global write "Robot Global Data.vi" "X axis"(w396) -> ()
          }
        }
      }
      frame Enabled {
      }
    }
    n268 = global read "Robot Global Data.vi" "Shoot"() -> (w373:bool)
    n269 = disable-structure shown="Enabled" {
      disable-tunnel: w382 -> [w411 _]
      disable-tunnel: w381 -> [w410 _]
      frame Enabled {
        n270 = global read "Robot Global Data.vi" "Servo"() -> (w409:i32)
        n271 = call <vilib>:"WPI_ServoSetAngle.vi"("Angle"=w409, "ServoDeviceRef"=w411) -> ()  [unwired: 8 in, 2 out]
        n272 = call <vilib>:"WPI_ServoSetAngle.vi"("Angle"=w409, "ServoDeviceRef"=w410) -> ()  [unwired: 8 in, 2 out]
      }
      frame Disabled {
      }
    }
    n273 = call <vilib>:"WPI_JoystickGet.vi"("JoystickDevRef"=w383) -> ("Buttons"=w380:T23)  [unwired: 1 in, 5 out]
    n274 = global read "Robot Global Data.vi" "turretSpeed"() -> (w375:dbl)
    n275 = disable-structure shown="Disabled" {
      disable-tunnel: w384 -> [w403 _]
      frame Disabled {
        n276 = call <vilib>:"WPI_GyroGetAngle.vi"("GyroDevRef"=w403) -> ("Angle"=w402:dbl)  [unwired: 7 in, 3 out]
        n277 = global write "Robot Global Data.vi" "Gyro Angle"(w402) -> ()
      }
      frame Enabled {
      }
    }
    n278 = Unbundle By Name(w380) -> ("Button 8"=w379:bool, "Button 9"=w378:bool, "Button 6"=w377:bool, "Button 7"=w374:bool)
    n279 = case shown="False" w379 {
      tunnel: w378 -> [w404 _]
      frame False {
        n280 = case shown="True" w404 {
          frame False {
          }
          frame True {
            n281 = global write "Robot Global Data.vi" "Servo"(124 ("Angle")) -> ()
            n282 = global write "Robot Global Data.vi" "Gear"(enum16{"Low Gear ", "None", "High Gear"}."High Gear" ("Gear")) -> ()
          }
        }
      }
      frame True {
        n283 = global write "Robot Global Data.vi" "Servo"(65 ("Angle")) -> ()
        n284 = global write "Robot Global Data.vi" "Gear"(enum16{"Low Gear ", "None", "High Gear"}."Low Gear " ("Gear")) -> ()
      }
    }
    n285 = case shown="False" w377 {
      tunnel: w374 -> [w398 _]
      tunnel: w373 -> [w397 _]
      frame False {
        n286 = case shown="False" w398 {
          tunnel: w397 -> [w399 _]
          frame False {
            n287 = case shown="False" w399 {
              frame False {
              }
              frame True {
              }
            }
          }
          frame True {
            n288 = global write "Robot Global Data.vi" "turretSpeed"(-0.5) -> ()
          }
        }
      }
      frame True {
        n289 = global write "Robot Global Data.vi" "turretSpeed"(0.5) -> ()
      }
    }
    n290 = call <vilib>:"WPI_MotorControlSetOutput.vi"("Output"=w375, "MotorControlDevRef"=w376) -> ()  [unwired: 7 in, 3 out]
    n291 = Wait (ms)(milliseconds to wait=u32 25) -> ()  [unwired: 1 out]
  }
  n292 = call <vilib>:"WPI_MotorControlRefNum Registry Get.vi"("refnum name"="Low Conveyor") -> ("MotorControlDevRef"=w13:T11)  [unwired: 9 in, 1 out]
  n293 = call <vilib>:"WPI_MotorControlRefNum Registry Get.vi"("refnum name"="Mid Conveyor") -> ("MotorControlDevRef"=w14:T11)  [unwired: 9 in, 1 out]
  n294 = call <vilib>:"WPI_MotorControlRefNum Registry Get.vi"("refnum name"="arm") -> ("MotorControlDevRef"=w15:T11)  [unwired: 9 in, 1 out]
  n295 = while {
    tunnel: w15 -> [w417]
    tunnel: w14 -> [w416]
    tunnel: w13 -> [w415]
    stop <- FALSE stop-if-true
    n296 = global read "Robot Global Data.vi" "Arm"() -> (w414:enum16{"Up", "Neutral", "Down"})
    n297 = global read "Robot Global Data.vi" "Bottom"() -> (w413:enum16{"Up", "Neutral", "Down"})
    n298 = global read "Robot Global Data.vi" "Middle"() -> (w412:enum16{"Up", "Neutral", "Down"})
    n299 = case shown="\"Neutral\", Default" w414 {
      tunnel: w417 -> [w433 w435 w436]
      frame "Up" {
        n300 = call <vilib>:"WPI_MotorControlSetOutput.vi"("Output"=1.0, "MotorControlDevRef"=w433) -> ()  [unwired: 7 in, 3 out]
      }
      frame "Neutral", Default {
        n301 = call <vilib>:"WPI_MotorControlSetOutput.vi"("Output"=0.0, "MotorControlDevRef"=w435) -> ()  [unwired: 7 in, 3 out]
      }
      frame "Down" {
        n302 = call <vilib>:"WPI_MotorControlSetOutput.vi"("Output"=-1.0, "MotorControlDevRef"=w436) -> ()  [unwired: 7 in, 3 out]
      }
    }
    n303 = case shown="\"Neutral\", Default" w413 {
      tunnel: w415 -> [w426 w429 w430]
      frame "Up" {
        n304 = call <vilib>:"WPI_MotorControlSetOutput.vi"("Output"=1.0, "MotorControlDevRef"=w426) -> ()  [unwired: 7 in, 3 out]
      }
      frame "Neutral", Default {
        n305 = call <vilib>:"WPI_MotorControlSetOutput.vi"("Output"=0.0, "MotorControlDevRef"=w429) -> ()  [unwired: 7 in, 3 out]
      }
      frame "Down" {
        n306 = call <vilib>:"WPI_MotorControlSetOutput.vi"("Output"=-1.0, "MotorControlDevRef"=w430) -> ()  [unwired: 7 in, 3 out]
      }
    }
    n307 = case shown="\"Neutral\", Default" w412 {
      tunnel: w416 -> [w420 w423 w424]
      frame "Up" {
        n308 = call <vilib>:"WPI_MotorControlSetOutput.vi"("Output"=1.0, "MotorControlDevRef"=w420) -> ()  [unwired: 7 in, 3 out]
      }
      frame "Neutral", Default {
        n309 = call <vilib>:"WPI_MotorControlSetOutput.vi"("Output"=0.0, "MotorControlDevRef"=w423) -> ()  [unwired: 7 in, 3 out]
      }
      frame "Down" {
        n310 = call <vilib>:"WPI_MotorControlSetOutput.vi"("Output"=-1.0, "MotorControlDevRef"=w424) -> ()  [unwired: 7 in, 3 out]
      }
    }
    n311 = Wait (ms)(milliseconds to wait=u32 50) -> ()  [unwired: 1 out]
  }
  n312 = while {
    stop <- FALSE stop-if-true
    # "This global is written to in the Autonomous and Teleop VIs"
    # "Flash the USER1 LED with the rate controlled from Autonomous and Teleop"
    n313 = global read "Robot Global Data.vi" "LED toggle rate (ms)"() -> (w438:u32)
    n314 = call <vilib>:"WPI_UtilitiesFRC LEDs.vi"("State"=FPGA_UtilitiesLED_State."Toggle", "LED Type"=FPGA_UtilitiesLED_Source."User LED") -> ()  [unwired: 1 in, 9 out]
    n315 = Wait (ms)(milliseconds to wait=w438) -> ()  [unwired: 1 out]
  }
